vi "SigleDotScale.vi"(9 "ScaleArray":dbl[][](array[numeric]), 10 "y":dbl=1.0, 11 "x":dbl=1.0) -> (1 "ScaleIndex":i32, 2 "y":dbl, 3 "x":dbl)   [LabVIEW 2011]
uses:
  <vilib>/vision/NI_Vision_Development_Module.lvlib
panel:
  out "floor(x): 最大整数 <= x":dbl
  out "floor(x/y)":sgl
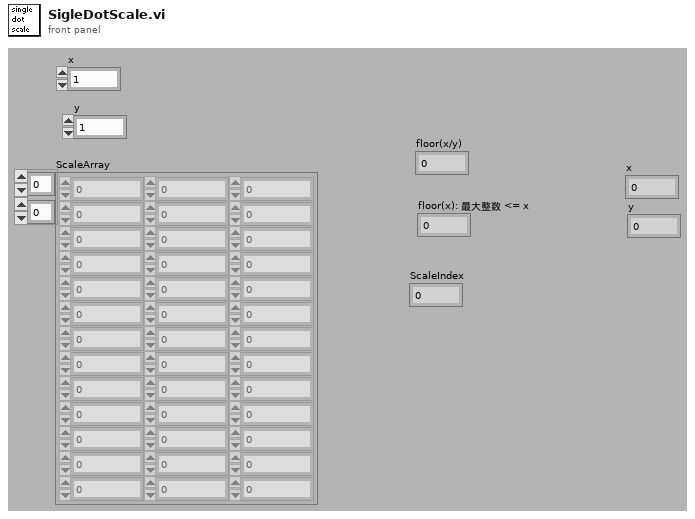
[diagram p1: front panel]
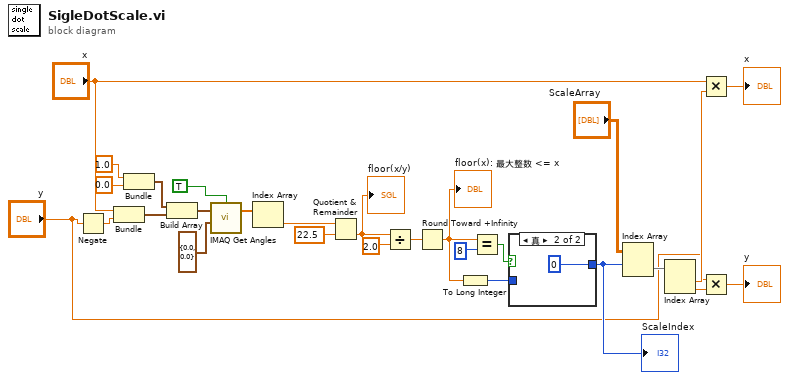
[diagram p0: block diagram]
diagram:
  n1 = Negate(x="y") -> (-x=w1:dbl)
  n2 = Bundle("x"="x", w1) -> (w25:cluster{"x":dbl, dbl})  [unwired: 1 out]
  n3 = Bundle(1.0, 0.0) -> (w24:cluster{dbl, dbl})  [unwired: 1 out]
  n4 = Build Array(w24, w25) -> (w23:cluster{"x":dbl, dbl}[])
  n5 = call "IMAQ Get Angles"("Vertex"=cluster{"X":sgl, "Y":sgl} {"X"=0.0, "Y"=0.0}, "Points"=w23, "Use Vertex (No)"=TRUE) -> ("Angles (deg)"=w20:sgl[])  [unwired: 1 in, 3 out]
  n6 = Index Array(array=w20) -> (element=w11:sgl)  [unwired: 1 in]
  n7 = Quotient & Remainder(x=w11, y=sgl 22.5) -> (floor(x/y)=w16:sgl)  [unwired: 1 out]
  "floor(x/y)" <- w16
  n8 = Divide(x=w16, y=2.0) -> (x/y=w18:dbl)
  n9 = Round Toward +Infinity(x=w18) -> (ceil(x): smallest int >= x=w13:dbl)
  "floor(x): 最大整数 <= x" <- w13
  n10 = To Long Integer(number=w13) -> (32bit integer=w12:i32)
  n11 = Equal?(x=w13, y=8) -> (x = y?=w14:bool)
  n12 = case shown="真" w14 {
    tunnel: [w28 0] -> w10
    tunnel: w12 -> [w28 _]
    frame False {
    }
    frame True {
    }
  }
  "ScaleIndex" <- w10
  n13 = Index Array(array="ScaleArray", index (row)=w10) -> (element=w8:dbl[])  [unwired: 1 in]
  n14 = Index Array(array=w8) -> (element #1=w7:dbl, element #2=w6:dbl)  [unwired: 2 in]
  n15 = Multiply(x="x", y=w7) -> (x*y=→"x":dbl)
  n16 = Multiply(x="y", y=w6) -> (x*y=→"y":dbl)
